vi "Project_Dream.vi"() -> ()   [LabVIEW 2022 SP3]
uses:
  53021927-9b32-4f58-bd55-e25aab92cb29.vi
  <vilib>/Instr/_visa.llb/VISA Configure Serial Port (Instr).vi
panel:
  out "Relay 7":bool
  out "Relay 6":bool
  out "Relay 5":bool
  out "Relay 4":bool
  out "Relay 3":bool
  out "Relay 2":bool
  out "Relay 1":bool
  out "Barth Connected?":bool
  out "read buffer":string
  in  "Message":string
  out "VISA resource out":refnum<visa-resource-name>
  in  "VISA resource in":refnum<visa-resource-name>
  in  "error in":errorcluster
  out "error out 2":errorcluster
  in  "1D Array":bool[](array[boolean])
  out "error out":errorcluster
  out "FTDI Connected?":bool
  out "FT_Status":u32(ring) items=["FT_OK", "FT_INVALID_HANDLE", "FT_DEVICE_NOT_FOUND", "FT_DEVICE_NOT_OPENED", "FT_IO_ERROR", "FT_INSUFFICIENT_RESOURCES", "FT_INVALID_PARAMETER", "FT_INVALID_BAUD_RATE", "FT_DEVICE_NOT_OPENED_FOR_ERASE", "FT_DEVICE_NOT_OPENED_FOR_WRITE", "FT_FAILED_TO_WRITE_DEVICE", "FT_EEPROM_READ_FAILED", "FT_EEPROM_WRITE_FAILED", "FT_EEPROM_ERASE_FAILED", "FT_EEPROM_NOT_PRESENT", "FT_EEPROM_NOT_PROGRAMMED", "FT_INVALID_ARGS", "FT_NOT_SUPPORTED", "FT_OTHER_ERROR"]
  out "Port Index":string
  out "Device Description":string
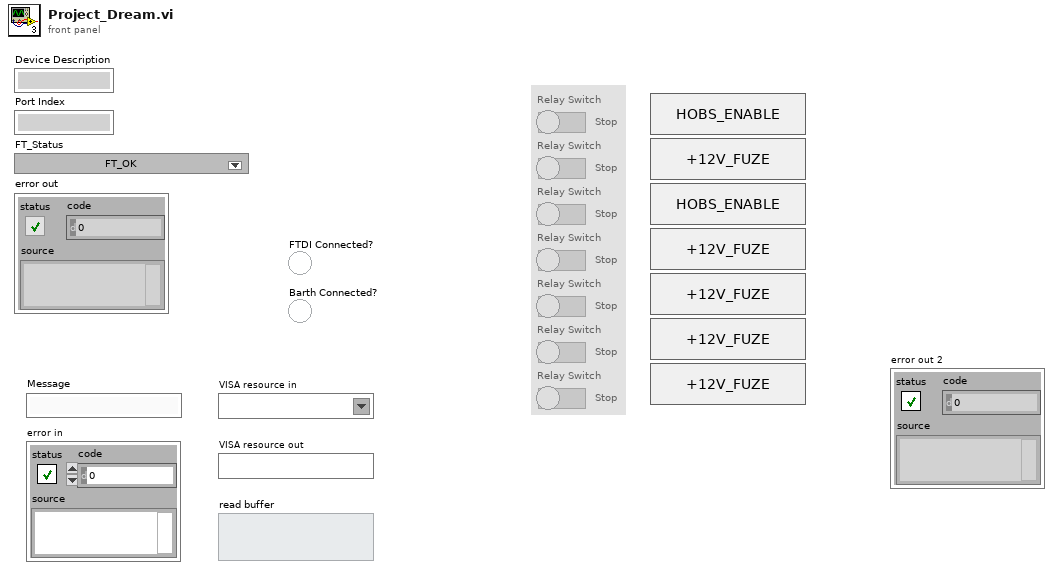
[diagram p1: front panel]
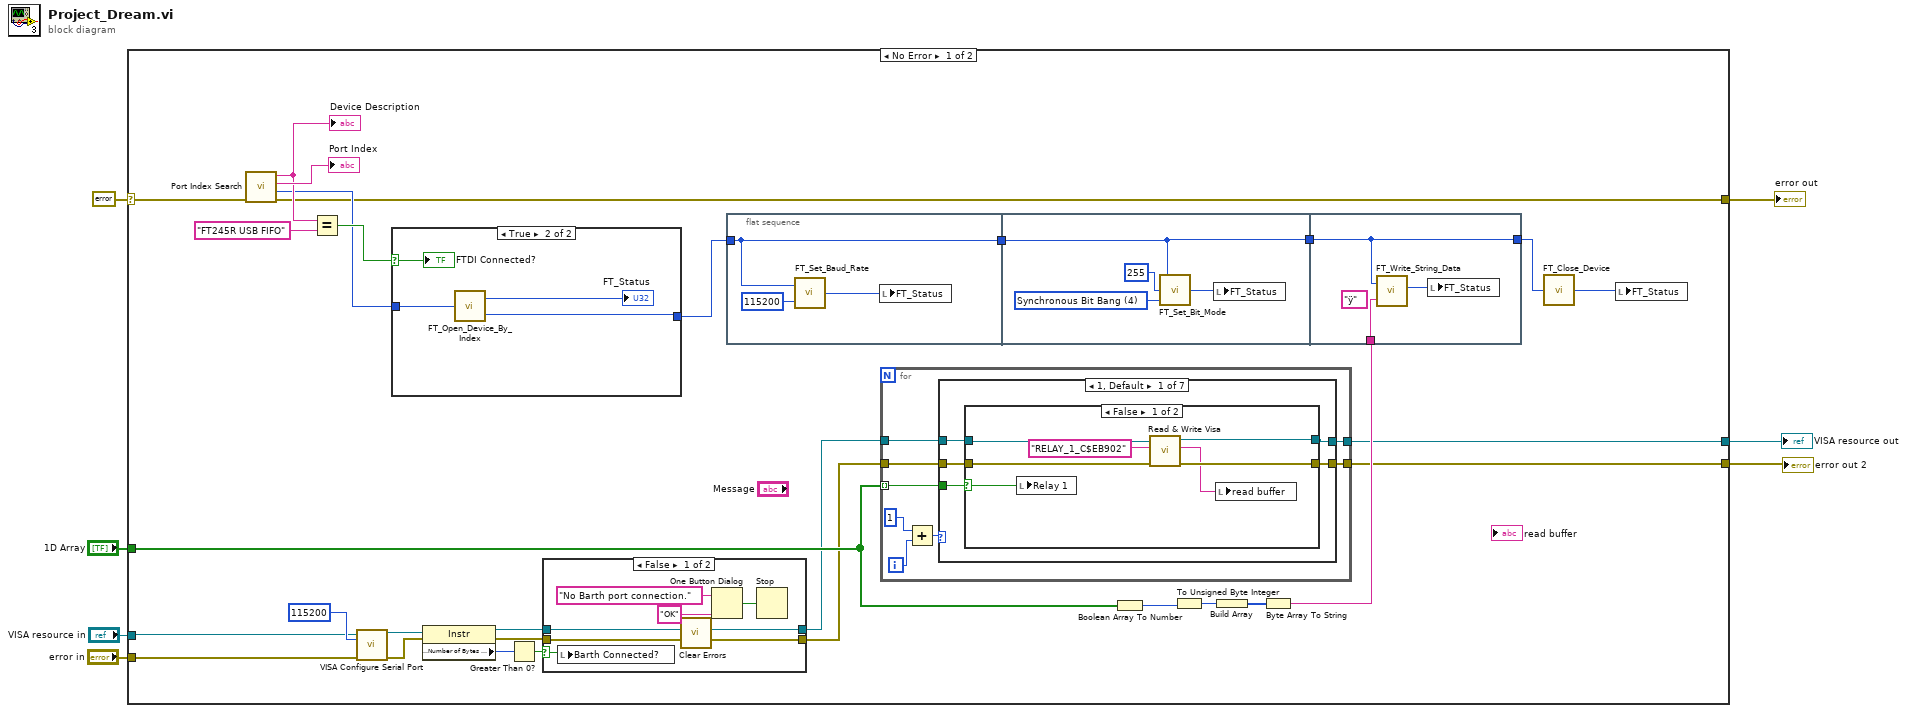
[diagram p0: block diagram]
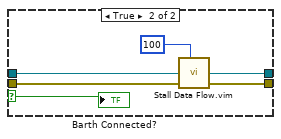
[diagram p2: hidden frame]
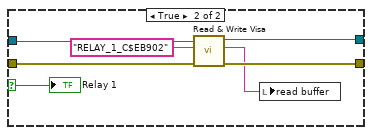
[diagram p3: hidden frame]
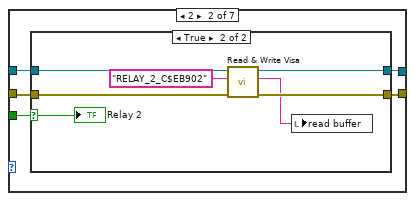
[diagram p4: hidden frame]
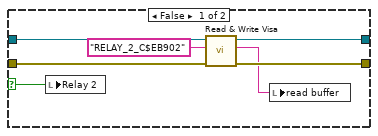
[diagram p5: hidden frame]
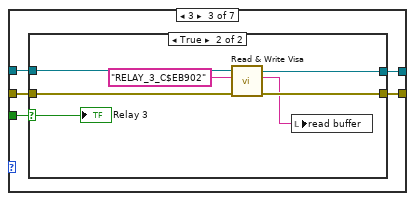
[diagram p6: hidden frame]
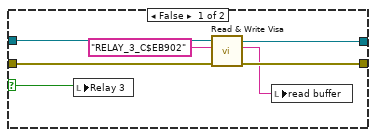
[diagram p7: hidden frame]
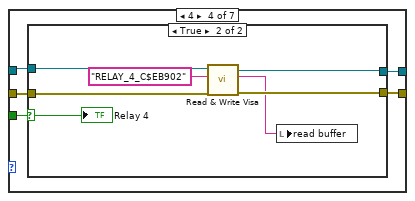
[diagram p8: hidden frame]
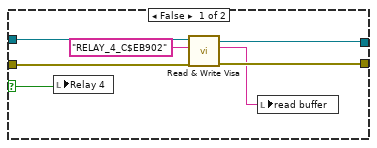
[diagram p9: hidden frame]
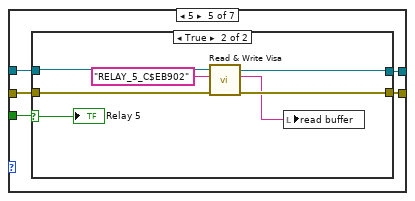
[diagram p10: hidden frame]
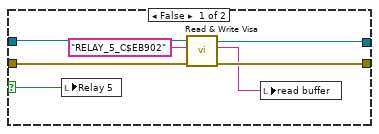
[diagram p11: hidden frame]
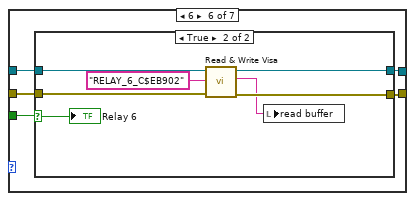
[diagram p12: hidden frame]
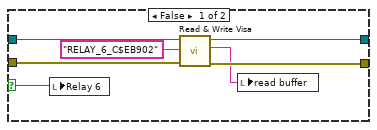
[diagram p13: hidden frame]
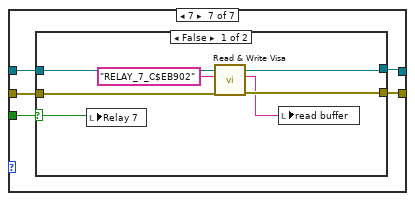
[diagram p14: hidden frame]
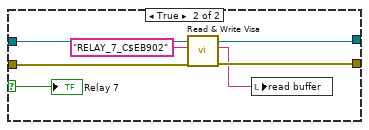
[diagram p15: hidden frame]
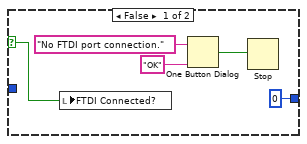
[diagram p16: hidden frame]
diagram:
  n1 = case shown="No Error" errorcluster {"status"=FALSE, "code"=0, "source"=""} ("error in") {
    selector: errorcluster {"status"=FALSE, "code"=0, "source"=""} ("error in") -> [w37 w212]
    tunnel: [w31 w212] -> w6
    tunnel: "1D Array" -> [w23 _]
    tunnel: "VISA resource in" -> [w21 w211]
    tunnel: "error in" -> [w20 w210]
    tunnel: [w11 w211] -> w2
    tunnel: [w10 w210] -> w1
    frame No Error {
      n2 = call "Port Index Search.vi"("error in"=w37) -> ("error out"=w31:errorcluster, "Decimal Port Index"=w32:i32, "Port Index"=→"Port Index":string, "Device Description"=w34:string)  [unwired: 7 in]
      "Device Description" <- w34
      n3 = Equal?(x=w34, y="FT245R USB FIFO") -> (x = y?=w33:bool)
      n4 = call-poly "VISA Configure Serial Port"("VISA resource name"=w21, "baud rate (9600)"=u32 115200 ("Baud Rate"), "error in (no error)"=w20) -> ("VISA resource name out"=w19:refnum<visa-resource-name>, "error out"=w18:errorcluster)  [unwired: 11 in]
      n5 = case shown="True" w33 {
        selector: w33 -> [w201 w207]
        tunnel: w32 -> [_ w209]
        tunnel: [0 ("Handle") w206] -> w30
        frame False {
          n6 = local write "FTDI Connected?"(w201) -> ()
          n7 = One Button Dialog(message="No FTDI port connection.", button name ("OK")="OK") -> (true=w202:bool)
          n8 = Stop(stop? (T)=w202) -> ()
        }
        frame True {
          n9 = call "FT_Open_Device_By_Index.vi"("Device Index"=w209) -> ("FT_Status"=→"FT_Status":u32, "Handle"=w206:i32)
          "FTDI Connected?" <- w207
        }
      }
      n10 = property class="Instr"(reference=w19, error in=w18) -> (reference out=w15:refnum<visa-resource-name>, error out=w14:errorcluster, "Serial Settings:Number of Bytes at Serial Port"=w17:u32)
      n11 = Greater Than 0?(x=w17) -> (x > 0?=w16:bool)
      n12 = case shown="False" w16 {
        selector: w16 -> [w38 w47]
        tunnel: w15 -> [w43 w49]
        tunnel: w14 -> [w42 w45]
        tunnel: [w43 w46] -> w13
        tunnel: [w41 w45] -> w12
        frame False {
          n13 = local write "Barth Connected?"(w38) -> ()
          n14 = call <vilib>:"Clear Errors.vi"("error in (no error)"=w42) -> ("error out"=w41:errorcluster)  [unwired: 5 in, 1 out]
          n15 = One Button Dialog(message="No Barth port connection.", button name ("OK")="OK") -> (true=w40:bool)
          n16 = Stop(stop? (T)=w40) -> ()
        }
        frame True {
          n17 = call "Stall Data Flow.vim"("value in"=w49, "milliseconds to wait"=u32 100) -> ("value out"=w46:refnum<visa-resource-name>)  [unwired: 1 out]
          "Barth Connected?" <- w47
        }
      }
      n18 = flat-sequence {
        tunnel: w30 -> [w191]
        tunnel: [w191] -> w29
        tunnel: w29 -> [w194]
        tunnel: [w194] -> w28
        tunnel: w28 -> [w199]
        tunnel: w27 -> [w198]
        tunnel: [w199] -> w8
        frame #0 {
          n19 = call "FT_Set_Baud_Rate.vi"("Baud Rate"=u32 115200, "Handle"=w191) -> ("FT_Status"=w192:u32)
          n20 = local write "FT_Status"(w192) -> ()
        }
        frame #1 {
          w196 = u8 4 items=["Reset Bit Mode"=0, "Asynchronous Bit Bang"=1, "MPSSE"=2, "Synchronous Bit Bang"=4, "MCU Host Bus Emulation"=8, "Fast Opto-Isolated Serial"=16, "CBUS Bit Bang"=32, "Single Channel 245 Synchronous FIFO"=64] ("Bit Mode")
          n21 = call "FT_Set_Bit_Mode.vi"("Bit Mode"=w196, "Bit Mode Mask"=u8 255, "Handle"=w194) -> ("FT_Status"=w195:u32)
          n22 = local write "FT_Status"(w195) -> ()
        }
        frame #2 {
          (unwired) "ÿ" ("Buffer")
          n23 = call "FT_Write_String_Data.vi"("Buffer"=w198, "Handle"=w199) -> ("FT_Status"=w200:u32)  [unwired: 1 out]
          n24 = local write "FT_Status"(w200) -> ()
        }
      }
      n25 = for {
        tunnel: w23 -> [w54] mode=indexing
        tunnel: w13 -> [w53]
        tunnel: w12 -> [w52]
        tunnel: [w51] -> w10
        tunnel: [w50] -> w11
        i -> [w56]
        n26 = Add(x=1, y=w56) -> (x+y=w55:i32)
        n27 = case shown="1, Default" w55 {
          tunnel: w54 -> [w62 w81 w100 w119 w138 w157 w176]
          tunnel: w53 -> [w61 w80 w99 w116 w137 w156 w174]
          tunnel: w52 -> [w60 w77 w98 w115 w136 w154 w175]
          tunnel: [w59 w78 w97 w118 w134 w153 w172] -> w51
          tunnel: [w58 w79 w96 w117 w135 w155 w173] -> w50
          frame 1, Default {
            n28 = case shown="False" w62 {
              selector: w62 -> [w63 w70]
              tunnel: w61 -> [w69 w76]
              tunnel: w60 -> [w68 w75]
              tunnel: [w66 w73] -> w58
              tunnel: [w65 w72] -> w59
              frame False {
                n29 = local write "Relay 1"(w63) -> ()
                n30 = call "Read & Write Visa.vi"("error in (no error)"=w68, "Message"="RELAY_1_C$EB902", "VISA Refnum in"=w69) -> ("error out"=w65:errorcluster, "read buffer"=w64:string, "VISA Refnum out"=w66:refnum<visa-resource-name>)  [unwired: 6 in]
                n31 = local write "read buffer"(w64) -> ()
              }
              frame True {
                n32 = call "Read & Write Visa.vi"("error in (no error)"=w75, "Message"="RELAY_1_C$EB902", "VISA Refnum in"=w76) -> ("error out"=w72:errorcluster, "read buffer"=w71:string, "VISA Refnum out"=w73:refnum<visa-resource-name>)  [unwired: 6 in]
                n33 = local write "read buffer"(w71) -> ()
                "Relay 1" <- w70
              }
            }
          }
          frame 2 {
            n34 = case shown="True" w81 {
              selector: w81 -> [w82 w90]
              tunnel: w80 -> [w88 w95]
              tunnel: [w87 w94] -> w79
              tunnel: [w86 w93] -> w78
              tunnel: w77 -> [w85 w92]
              frame False {
                n35 = local write "Relay 2"(w82) -> ()
                n36 = call "Read & Write Visa.vi"("error in (no error)"=w85, "Message"="RELAY_2_C$EB902", "VISA Refnum in"=w88) -> ("error out"=w86:errorcluster, "read buffer"=w83:string, "VISA Refnum out"=w87:refnum<visa-resource-name>)  [unwired: 6 in]
                n37 = local write "read buffer"(w83) -> ()
              }
              frame True {
                n38 = call "Read & Write Visa.vi"("error in (no error)"=w92, "Message"="RELAY_2_C$EB902", "VISA Refnum in"=w95) -> ("error out"=w93:errorcluster, "read buffer"=w89:string, "VISA Refnum out"=w94:refnum<visa-resource-name>)  [unwired: 6 in]
                n39 = local write "read buffer"(w89) -> ()
                "Relay 2" <- w90
              }
            }
          }
          frame 3 {
            n40 = case shown="True" w100 {
              selector: w100 -> [w101 w108]
              tunnel: w99 -> [w107 w114]
              tunnel: w98 -> [w105 w112]
              tunnel: [w104 w111] -> w97
              tunnel: [w103 w110] -> w96
              frame False {
                n41 = local write "Relay 3"(w101) -> ()
                n42 = call "Read & Write Visa.vi"("error in (no error)"=w105, "Message"="RELAY_3_C$EB902", "VISA Refnum in"=w107) -> ("error out"=w104:errorcluster, "read buffer"=w102:string, "VISA Refnum out"=w103:refnum<visa-resource-name>)  [unwired: 6 in]
                n43 = local write "read buffer"(w102) -> ()
              }
              frame True {
                n44 = call "Read & Write Visa.vi"("error in (no error)"=w112, "Message"="RELAY_3_C$EB902", "VISA Refnum in"=w114) -> ("error out"=w111:errorcluster, "read buffer"=w109:string, "VISA Refnum out"=w110:refnum<visa-resource-name>)  [unwired: 6 in]
                n45 = local write "read buffer"(w109) -> ()
                "Relay 3" <- w108
              }
            }
          }
          frame 4 {
            n46 = case shown="True" w119 {
              selector: w119 -> [w120 w127]
              tunnel: [w126 w133] -> w118
              tunnel: [w125 w132] -> w117
              tunnel: w116 -> [w124 w131]
              tunnel: w115 -> [w123 w130]
              frame False {
                n47 = local write "Relay 4"(w120) -> ()
                n48 = call "Read & Write Visa.vi"("error in (no error)"=w123, "Message"="RELAY_4_C$EB902", "VISA Refnum in"=w124) -> ("error out"=w126:errorcluster, "read buffer"=w121:string, "VISA Refnum out"=w125:refnum<visa-resource-name>)  [unwired: 6 in]
                n49 = local write "read buffer"(w121) -> ()
              }
              frame True {
                n50 = call "Read & Write Visa.vi"("error in (no error)"=w130, "Message"="RELAY_4_C$EB902", "VISA Refnum in"=w131) -> ("error out"=w133:errorcluster, "read buffer"=w128:string, "VISA Refnum out"=w132:refnum<visa-resource-name>)  [unwired: 6 in]
                n51 = local write "read buffer"(w128) -> ()
                "Relay 4" <- w127
              }
            }
          }
          frame 5 {
            n52 = case shown="True" w138 {
              selector: w138 -> [w139 w146]
              tunnel: w137 -> [w145 w152]
              tunnel: w136 -> [w144 w151]
              tunnel: [w143 w150] -> w135
              tunnel: [w142 w149] -> w134
              frame False {
                n53 = local write "Relay 5"(w139) -> ()
                n54 = call "Read & Write Visa.vi"("error in (no error)"=w144, "Message"="RELAY_5_C$EB902", "VISA Refnum in"=w145) -> ("error out"=w142:errorcluster, "read buffer"=w140:string, "VISA Refnum out"=w143:refnum<visa-resource-name>)  [unwired: 6 in]
                n55 = local write "read buffer"(w140) -> ()
              }
              frame True {
                n56 = call "Read & Write Visa.vi"("error in (no error)"=w151, "Message"="RELAY_5_C$EB902", "VISA Refnum in"=w152) -> ("error out"=w149:errorcluster, "read buffer"=w147:string, "VISA Refnum out"=w150:refnum<visa-resource-name>)  [unwired: 6 in]
                n57 = local write "read buffer"(w147) -> ()
                "Relay 5" <- w146
              }
            }
          }
          frame 6 {
            n58 = case shown="True" w157 {
              selector: w157 -> [w158 w165]
              tunnel: w156 -> [w164 w171]
              tunnel: [w163 w170] -> w155
              tunnel: w154 -> [w162 w169]
              tunnel: [w161 w168] -> w153
              frame False {
                n59 = local write "Relay 6"(w158) -> ()
                n60 = call "Read & Write Visa.vi"("error in (no error)"=w162, "Message"="RELAY_6_C$EB902", "VISA Refnum in"=w164) -> ("error out"=w161:errorcluster, "read buffer"=w159:string, "VISA Refnum out"=w163:refnum<visa-resource-name>)  [unwired: 6 in]
                n61 = local write "read buffer"(w159) -> ()
              }
              frame True {
                n62 = call "Read & Write Visa.vi"("error in (no error)"=w169, "Message"="RELAY_6_C$EB902", "VISA Refnum in"=w171) -> ("error out"=w168:errorcluster, "read buffer"=w166:string, "VISA Refnum out"=w170:refnum<visa-resource-name>)  [unwired: 6 in]
                n63 = local write "read buffer"(w166) -> ()
                "Relay 6" <- w165
              }
            }
          }
          frame 7 {
            n64 = case shown="False" w176 {
              selector: w176 -> [w177 w184]
              tunnel: w175 -> [w183 w190]
              tunnel: w174 -> [w182 w189]
              tunnel: [w181 w188] -> w173
              tunnel: [w180 w187] -> w172
              frame False {
                n65 = local write "Relay 7"(w177) -> ()
                n66 = call "Read & Write Visa.vi"("error in (no error)"=w183, "Message"="RELAY_7_C$EB902", "VISA Refnum in"=w182) -> ("error out"=w180:errorcluster, "read buffer"=w178:string, "VISA Refnum out"=w181:refnum<visa-resource-name>)  [unwired: 6 in]
                n67 = local write "read buffer"(w178) -> ()
              }
              frame True {
                n68 = call "Read & Write Visa.vi"("error in (no error)"=w190, "Message"="RELAY_7_C$EB902", "VISA Refnum in"=w189) -> ("error out"=w187:errorcluster, "read buffer"=w185:string, "VISA Refnum out"=w188:refnum<visa-resource-name>)  [unwired: 6 in]
                n69 = local write "read buffer"(w185) -> ()
                "Relay 7" <- w184
              }
            }
          }
        }
      }
      n70 = Boolean Array To Number(Boolean array=w23) -> (number=w24:u32)
      n71 = To Unsigned Byte Integer(number=w24) -> (unsigned 8bit integer=w25:u8)
      n72 = Build Array(w25) -> (w26:u8[])
      n73 = Byte Array To String(unsigned byte array=w26) -> (string=w27:string)
      n74 = call "FT_Close_Device.vi"("Handle"=w8) -> ("FT_Status"=w9:u32)
      n75 = local write "FT_Status"(w9) -> ()
    }
    frame Error {
    }
  }
  "error out" <- w6
  "error out 2" <- w1
  "VISA resource out" <- w2
